vi "Set Scan Settings.vi"(10 "Test Settings":T1 {"Lateral Load Cell Sensitivity" format="%.6f"; "Axial Load Cell Sensitivity" format="%.6f"}, 11 "Model in":refnum<class "Model.lvclass">) -> (3 "Model out":refnum<class "Model.lvclass">)   [LabVIEW 2015, in "Model.lvclass"]
uses:
  Model.lvclass
  Typedefs/TestSettings.ctl
  Common_RT_FAILC/DataTypes/FATypes.ctl
  Model.lvclass/Model.ctl
  Typedefs/FAMT Typedefs.lvlib
  Common_RT_FAILC/RTFAILC.lvlib
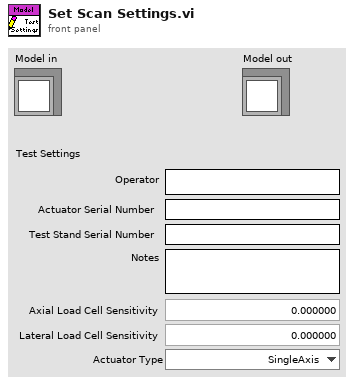
[diagram p1: front panel]
types:
  T1 = typedef "FAMT Typedefs.lvlib/TestSettings.ctl" = cluster{"Operator":string, "Notes":string, "Actuator Serial Number":string, "Test Stand Serial Number":string, "Axial Load Cell Sensitivity":dbl, "Lateral Load Cell Sensitivity":dbl, "Actuator Type":T2}
  T2 = typedef "RTFAILC.lvlib/FATypes.ctl" = enum16{"SingleAxis", "LateralDualAxis", "CrossLateralDualAxis"}
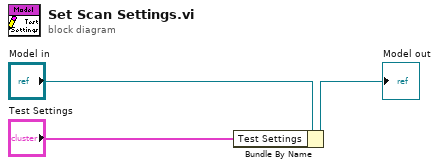
[diagram p0: block diagram]
diagram:
  n1 = Bundle By Name(cluster="Model in", "Test Settings"="Test Settings") -> (→"Model out":refnum<class "Model.lvclass">)
